vi "Translational motor output.vi"(0 "Command":T1(ring)=enum."Manual", 1 "motor 1 angle":dbl=30.0, 2 "motor 2 angle":dbl=150.0, 3 "motor 3 angle":dbl=270.0, 4 "motor 4 angle":dbl, 5 "error in":errorcluster, 6 "manual input angle":dbl=90.0, 7 "Trans spd multiplier":dbl=1.0, 8 "Orientation":dbl) -> (15 "motor 1 out":dbl=1.0 format="%#.4f", 16 "motor 2 out":dbl format="%#.4f", 17 "motor 3 out":dbl=1.2246467991473532e-16 format="%#.4f", 18 "motor 4 out":dbl=-1.0 format="%#.4f", 19 "error out":errorcluster)   [LabVIEW 2017]
panel:
  out "motor 4\nspeed multiplier":dbl=-1.0 format="%#.4f"
  out "motor 3\nspeed multiplier":dbl=1.2246467991473532e-16 format="%#.4f"
  out "motor 2\nspeed multiplier":dbl format="%#.4f"
  out "motor 1\nspeed multiplier":dbl=1.0 format="%#.4f"
  # "VI Description: Calculates the desired outputs for each motor given a direction to move and the robot's current orientation"
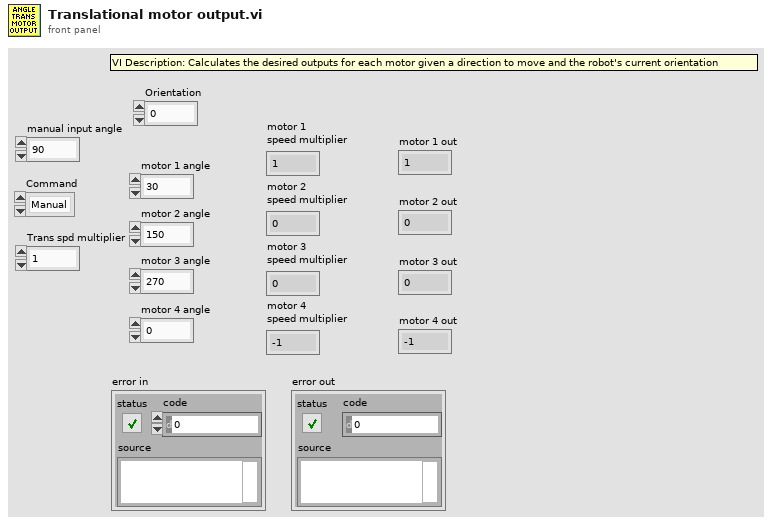
[diagram p1: front panel]
types:
  T1 = enum16{"Stop / None", "Forward", "Backward", "Left", "Right", "Manual"}
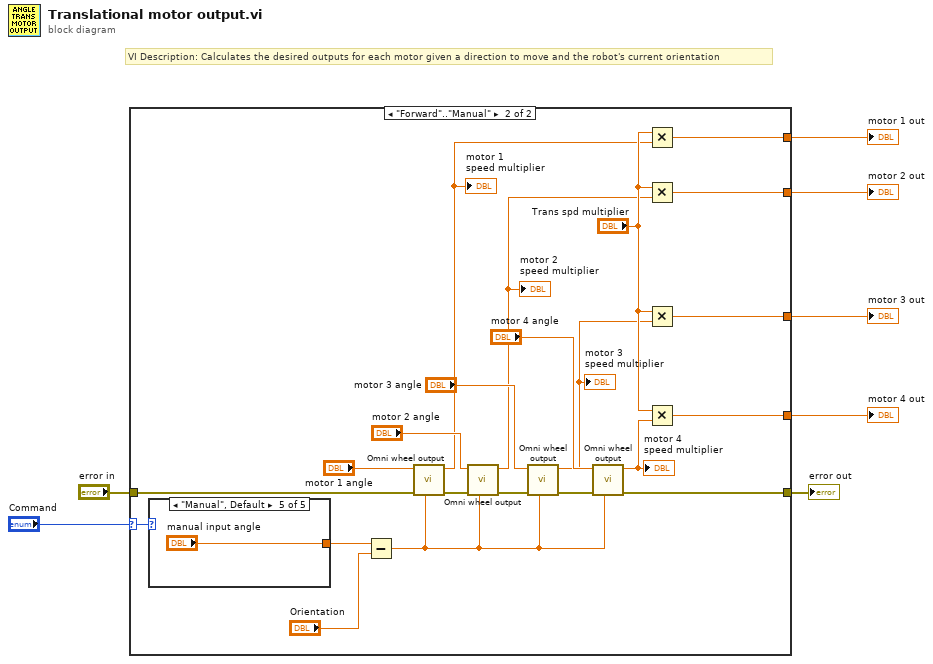
[diagram p0: block diagram]
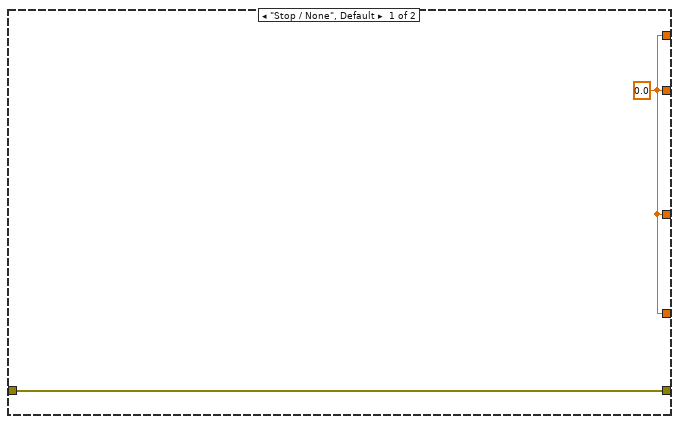
[diagram p2: hidden frame]
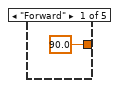
[diagram p3: hidden frame]
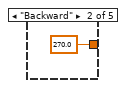
[diagram p4: hidden frame]
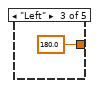
[diagram p5: hidden frame]
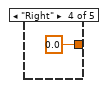
[diagram p6: hidden frame]
diagram:
  # "VI Description: Calculates the desired outputs for each motor given a direction to move and the robot's current orientation"
  n1 = case shown="\"Forward\"..\"Manual\"" "Command" {
    selector: "Command" -> [_ w27]
    tunnel: [w9 w22] -> w7
    tunnel: [w9 w21] -> w6
    tunnel: [w9 w20] -> w5
    tunnel: [w9 w19] -> w4
    tunnel: "error in" -> [w8 w17]
    tunnel: [w8 w13] -> w1
    frame "Stop / None", Default {
      w9 = 0.0
    }
    frame "Forward".."Manual" {
      n2 = case shown="\"Manual\", Default" w27 {
        tunnel: [90.0 270.0 ("input angle") 180.0 ("input angle") 0.0 ("input angle") "manual input angle"] -> w11
        frame "Forward" {
        }
        frame "Backward" {
        }
        frame "Left" {
        }
        frame "Right" {
        }
        frame "Manual", Default {
        }
      }
      n3 = Subtract(x=w11, y="Orientation") -> (x-y=w10:dbl)
      n4 = call "Omni wheel output.vi"("input angle"=w10, "error in"=w17, "motor angle"="motor 1 angle") -> ("error out"=w16:errorcluster, "speed multiplier"=w25:dbl)  [unwired: 7 in]
      "motor 1\nspeed multiplier" <- w25
      n5 = call "Omni wheel output.vi"("input angle"=w10, "error in"=w16, "motor angle"="motor 2 angle") -> ("error out"=w15:errorcluster, "speed multiplier"=w24:dbl)  [unwired: 7 in]
      "motor 2\nspeed multiplier" <- w24
      n6 = call "Omni wheel output.vi"("input angle"=w10, "error in"=w15, "motor angle"="motor 3 angle") -> ("error out"=w14:errorcluster, "speed multiplier"=w23:dbl)  [unwired: 7 in]
      "motor 3\nspeed multiplier" <- w23
      n7 = call "Omni wheel output.vi"("input angle"=w10, "error in"=w14, "motor angle"="motor 4 angle") -> ("error out"=w13:errorcluster, "speed multiplier"=w18:dbl)  [unwired: 7 in]
      "motor 4\nspeed multiplier" <- w18
      n8 = Multiply(x="Trans spd multiplier", y=w25) -> (x*y=w21:dbl)
      n9 = Multiply(x="Trans spd multiplier", y=w24) -> (x*y=w20:dbl)
      n10 = Multiply(x="Trans spd multiplier", y=w23) -> (x*y=w19:dbl)
      n11 = Multiply(x="Trans spd multiplier", y=w18) -> (x*y=w22:dbl)
    }
  }
  "motor 1 out" <- w6
  "motor 2 out" <- w5
  "motor 3 out" <- w4
  "motor 4 out" <- w7
  "error out" <- w1
